vi "vision.vi"(8 "error in":errorcluster, 11 "Image In":T2) -> (0 "error out":errorcluster, 2 "Shape Report (Shape Matching 1)":T3(array[cluster]) {"Score" format="%.2f"; "Centroid"."y" format="%.2f"; "Centroid"."x" format="%.2f"}, 3 "Image Out":T2)   [LabVIEW 2015]
uses:
  <vilib>/vision/Image Controls.llb/IMAQ Image.ctl
  <vilib>/vision/NI_Vision_Development_Module.lvlib
panel:
  out "Coordinate System Out (Set Coordinate System 1)":T1 {"Measurement System"."Axis Reference" items=["Direct", "Indirect"]; "Measurement System"."Angle (deg)" format="%.2f"; "Measurement System"."Origin"."Y" format="%.2f"; "Measurement System"."Origin"."X" format="%.2f"; "Reference System"."Axis Reference" items=["Direct", "Indirect"]; "Reference System"."Angle (deg)" format="%.2f"; "Reference System"."Origin"."Y" format="%.2f"; "Reference System"."Origin"."X" format="%.2f"}
  out "Shape Report (calibrated) (Shape Matching 1)":T3(array[cluster]) {"Score" format="%.2f"; "Centroid"."y" format="%.2f"; "Centroid"."x" format="%.2f"}
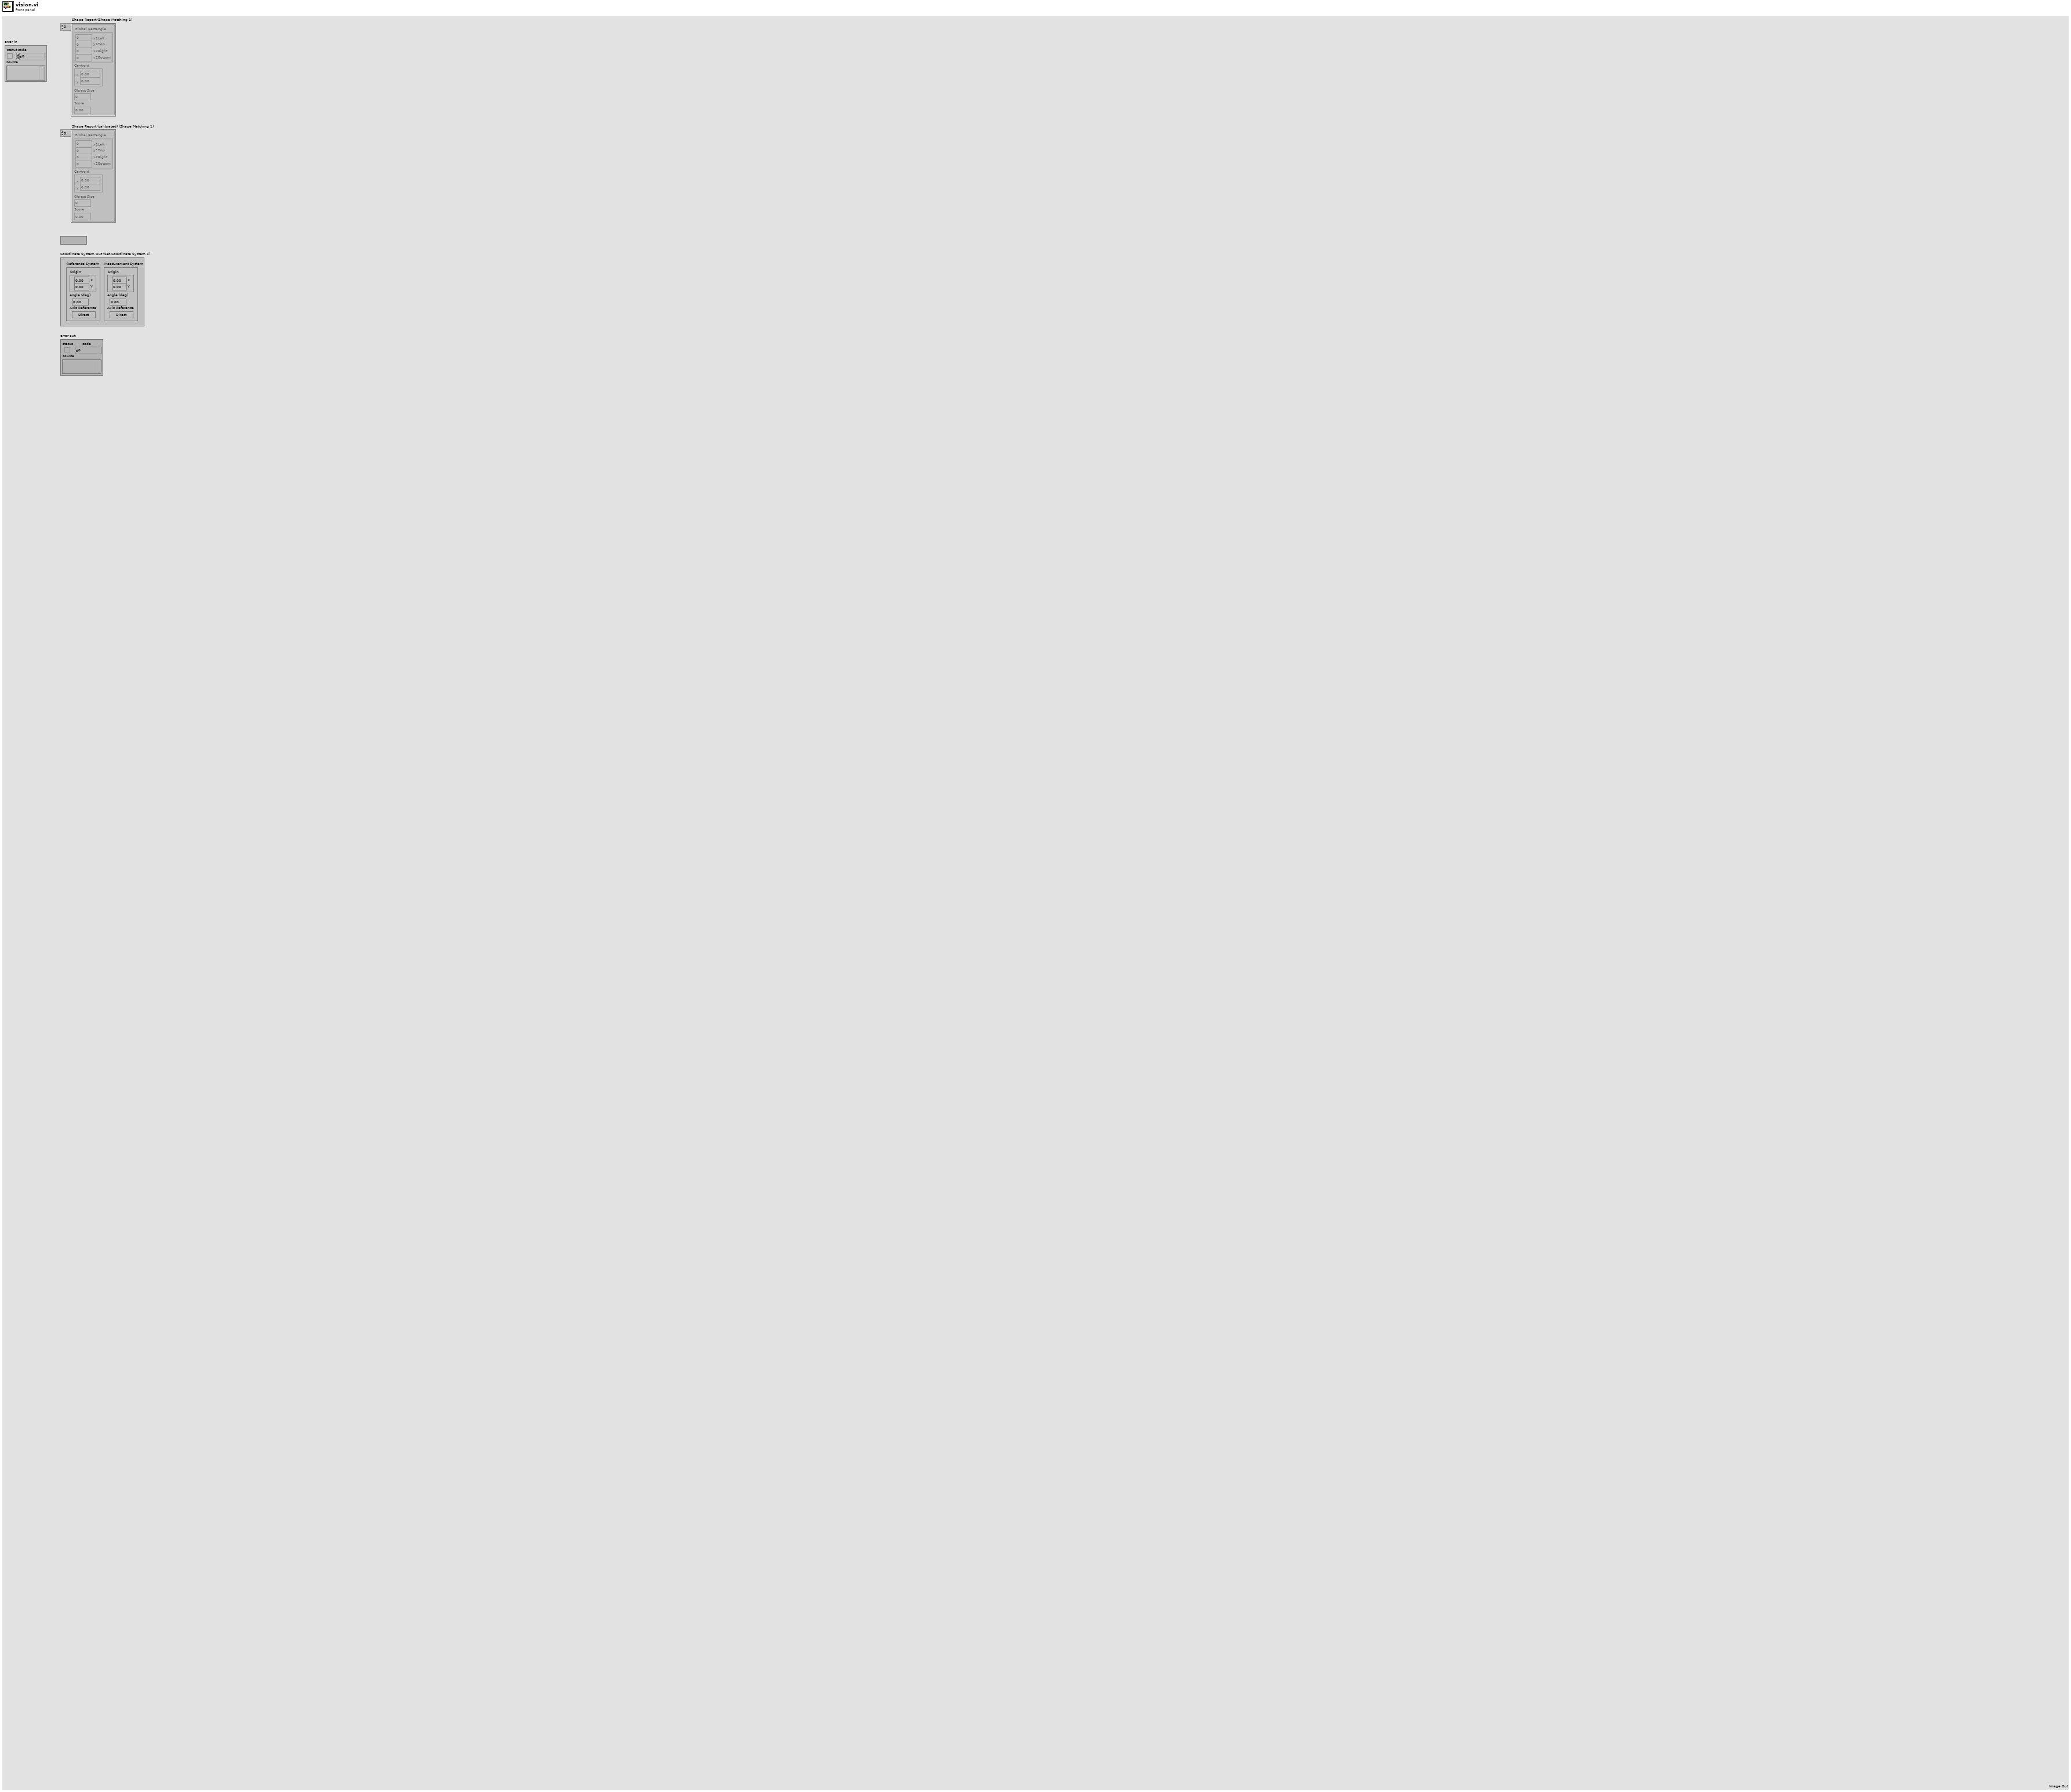
[diagram p1: front panel]
types:
  T1 = cluster{"Reference System":cluster{"Origin":cluster{"X":sgl, "Y":sgl}, "Angle (deg)":sgl, "Axis Reference":u32}, "Measurement System":cluster{"Origin":cluster{"X":sgl, "Y":sgl}, "Angle (deg)":sgl, "Axis Reference":u32}}
  T2 = typedef "IMAQ Image.ctl" = refnum<image>
  T3 = cluster{"Global Rectangle":cluster{"x1Left":i32, "y1Top":i32, "x2Right":i32, "y2Bottom":i32}, "Centroid":cluster{"x":sgl, "y":sgl}, "Object Size":u32, "Score":dbl}[]
  T4 = enum16{"Reset", "Update Coordinate System", "Get Coordinate System"}
  T5 = enum16{"Horizontal Motion", "Vertical Motion", "Horizontal and Vertical Motion", "Horizontal, Vertical and Angular Motion"}
  T6 = cluster{"Origin":cluster{"X":sgl, "Y":sgl}, "Angle (deg)":sgl, "Axis Reference":u32}
  T7 = typedef "IMAQ Coordinate System" = cluster{"Reference System":cluster{"Origin":cluster{"X":sgl, "Y":sgl}, "Angle (deg)":sgl, "Axis Reference":u32}, "Measurement System":cluster{"Origin":cluster{"X":sgl, "Y":sgl}, "Angle (deg)":sgl, "Axis Reference":u32}}
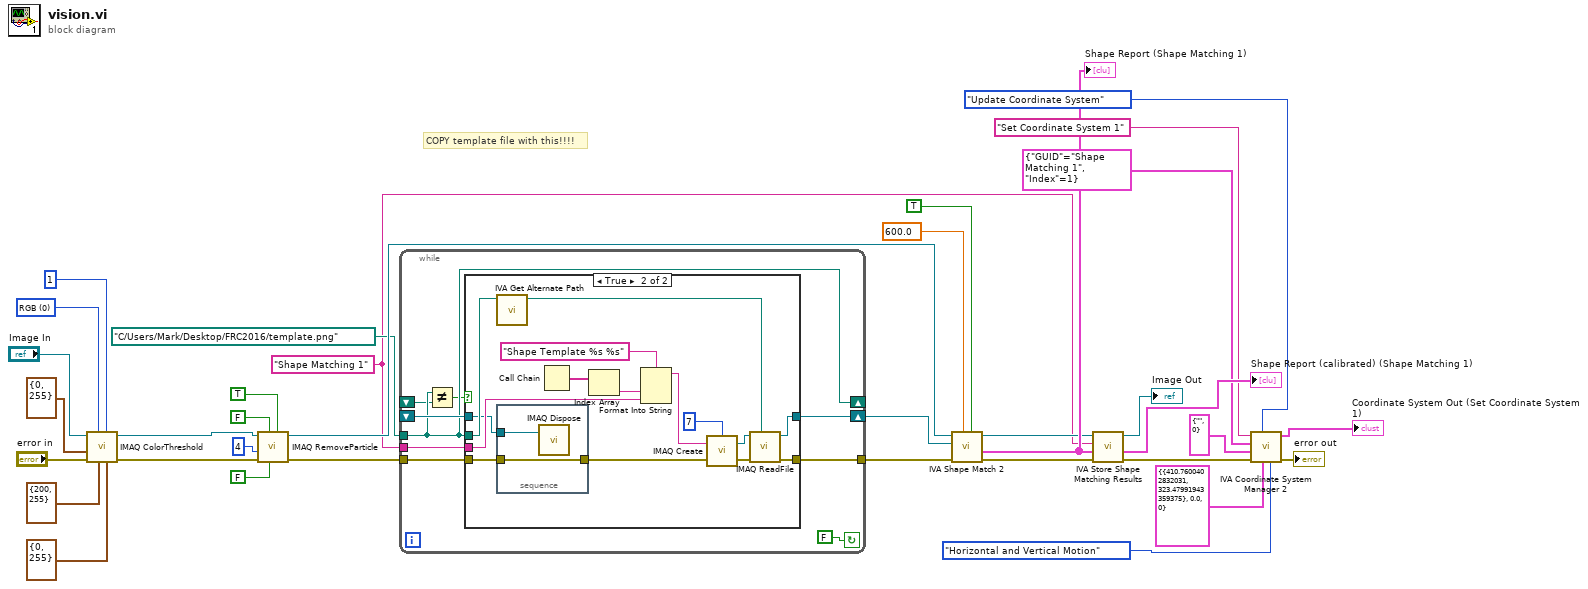
[diagram p0: block diagram]
diagram:
  w11 = "Shape Matching 1" ("Step Name")
  w34 = u16 0 items=["RGB", "HSL", "HSV", "HSI"] ("Color Mode")
  # "COPY template file with this!!!!"
  n1 = call "IMAQ ColorThreshold"("Blue or Luma or Val or Inten Range"=cluster{"Lower value":i32, "Upper value":i32} {"Lower value"=0, "Upper value"=255}, "Replace Value"=1, "Green or Sat Range"=cluster{"Lower value":i32, "Upper value":i32} {"Lower value"=200, "Upper value"=255}, "Color Mode"=w34, "error in (no error)"="error in", "Red or Hue Range"=cluster{"Lower value":i32, "Upper value":i32} {"Lower value"=0, "Upper value"=255}, "Image Src"="Image In") -> ("error out"=w23:errorcluster, "Image Dst Out"=w24:T2)  [unwired: 1 in, 2 out]
  n2 = call "IMAQ RemoveParticle"("Connectivity 4/8 (8)"=TRUE, "Low Pass/High Pass (Low)"=FALSE, "Square/Hexa (Square)"=FALSE, "error in (no error)"=w23, "Number of Erosion"=4, "Image Src"=w24) -> ("error out"=w14:errorcluster, "Image Dst Out"=w20:T2)  [unwired: 1 in, 3 out]
  n3 = while {
    shift-right: [w44] -> w12
    shift-left: _ -> [w43]
    tunnel: [w41] -> w13
    tunnel: w14 -> [w40]
    tunnel: path "C:/Users/Mark/Desktop/FRC2016/template.png" ("Template Path") -> [w38]
    tunnel: w11 -> [w39]
    shift-right: [w38] -> _
    shift-left: _ -> [w37]
    stop <- FALSE continue-if-true
    n4 = Not Equal?(x=w38, y=w37) -> (x != y?=w36:bool)
    n5 = case shown="True" w36 {
      tunnel: [w46 w58] -> w44
      tunnel: w43 -> [w46 w49]
      tunnel: [w45 w56] -> w41
      tunnel: w40 -> [w45 w48]
      tunnel: w38 -> [_ w51]
      tunnel: w39 -> [_ w52]
      frame False {
      }
      frame True {
        n6 = call <vilib>:"IVA Get Alternate Path.vi"("Path In"=w51) -> ("Path Out"=w50:path)  [unwired: 10 out]
        n7 = stacked-sequence {
          tunnel: w49 -> [w63]
          tunnel: w48 -> [w62]
          tunnel: [w62] -> w47
          frame #0 {
            n8 = call "IMAQ Dispose"("Image"=w63) -> ()  [unwired: 2 in, 4 out]
          }
        }
        n9 = Call Chain() -> (call chain=w54:string[])
        n10 = Index Array(array=w54) -> (element=w53:string)  [unwired: 1 in]
        n11 = Format Into String(format string="Shape Template %s %s" ("Image Name"), w53, w52) -> (resulting string=w61:string)  [unwired: 2 in, 1 out]
        n12 = call "IMAQ Create"("Border Size"=7, "Image Name"=w61, "error in (no error)"=w47) -> ("New Image"=w59:T2, "error out"=w57:errorcluster)  [unwired: 1 in, 1 out]
        n13 = call "IMAQ ReadFile"("File Path"=w50, "error in (no error)"=w57, "Image"=w59) -> ("error out"=w56:errorcluster, "Image Out"=w58:T2)  [unwired: 2 in, 5 out]
      }
    }
  }
  n14 = call <vilib>:"IVA Shape Match 2.vi"("Scale Invariance"=TRUE, "Minimal Score"=600.0, "error in (no error)"=w13, "Template"=w12, "Image Src"=w20) -> ("error out"=w19:errorcluster, "Shape Report"=w18:T3, "Image Out"=w17:T2)  [unwired: 4 out]
  "Shape Report (Shape Matching 1)" <- w18
  n15 = call <vilib>:"IVA Store Shape Matching Results.vi"("error in (no error)"=w19, "Shape Report"=w18, "Step Name"=w11, "Image in"=w17) -> ("error out"=w3:errorcluster, "Shape Report (calibrated)"=→"Shape Report (calibrated) (Shape Matching 1)":T3, "Image dup"=→"Image Out":T2)  [unwired: 5 out]
  n16 = call <vilib>:"IVA Coordinate System Manager 2.vi"("Mode"=T5."Horizontal and Vertical Motion", "Reference System"=T6 {"Origin"={"X"=410.76004, "Y"=323.47992}, "Angle (deg)"=0.0, "Axis Reference"=0}, "Function"=T4."Update Coordinate System", "error in (no error)"=w3, "Angle ID"=cluster{"GUID":string, "Index":i32} {"GUID"="", "Index"=0}, "Origin ID"=cluster{"GUID":string, "Index":i32} {"GUID"="Shape Matching 1", "Index"=1}, "Coordinate System Name"="Set Coordinate System 1") -> ("error out"=→"error out":errorcluster, "Coordinate System Out"=→"Coordinate System Out (Set Coordinate System 1)":T7)  [unwired: 3 out]
